vi "Init.vi"(5 "Instrument.lvclass 2":refnum<class "Instrument.lvclass">, 6 "Step":dbl, 7 "Instrument 1.lvclass":refnum<class "Instrument.lvclass">, 8 "error in (no error)":errorcluster, 9 "Max":dbl, 10 "Init":dbl, 11 "Measurement1D in":refnum<class "Measurement2D.lvclass">) -> (0 "error out":errorcluster, 3 "Measurement1D out":refnum<class "Measurement2D.lvclass">)   [LabVIEW 2018, in "Measurement2D.lvclass"]
uses:
  Measurement2D.lvclass
  Instrument/Instrument/Instrument.lvclass
  Measurement2D.lvclass/Measurement2D.ctl
panel:
  in  "Current Value":dbl
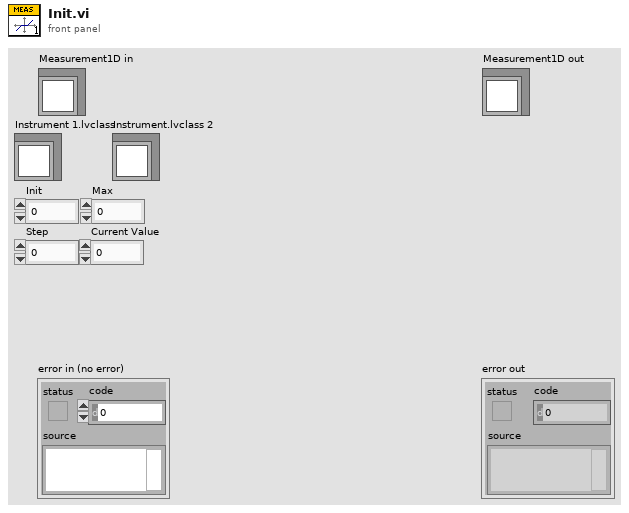
[diagram p1: front panel]
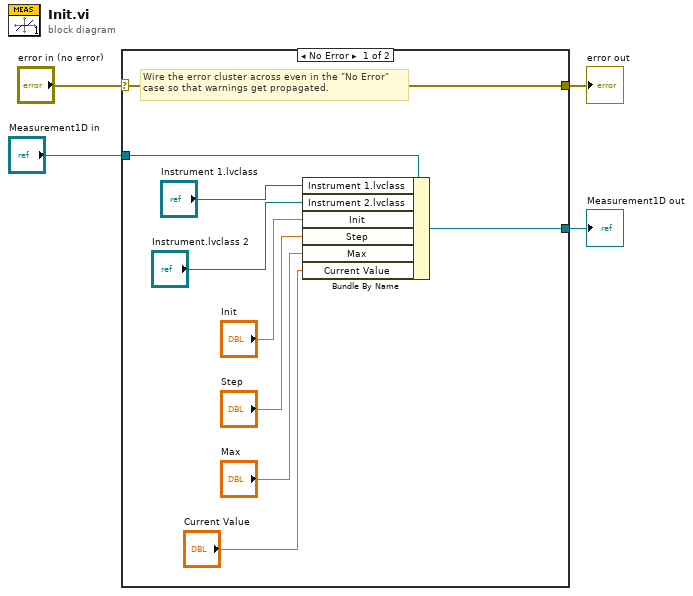
[diagram p0: block diagram]
diagram:
  n1 = case shown="No Error" "error in (no error)" {
    selector: "error in (no error)" -> [w13 w15]
    tunnel: [w13 w15] -> w3
    tunnel: [w5 w14] -> w1
    tunnel: "Measurement1D in" -> [w12 w14]
    frame No Error {
      # "Wire the error cluster across even in the \"No Error\"\ncase so that warnings get propagated."
      n2 = Bundle By Name(cluster=w12, "Instrument 1.lvclass"="Instrument 1.lvclass", "Instrument 2.lvclass"="Instrument.lvclass 2", "Init"="Init", "Step"="Step", "Max"="Max", "Current Value"="Current Value") -> (w5:refnum<class "Measurement2D.lvclass">)
    }
    frame Error {
    }
  }
  "error out" <- w3
  "Measurement1D out" <- w1
